vi "PSAS Data to text file (2).vi"(8 "Eixo":string, 9 "2nd column array":dbl[](array[numeric]), 10 "1st column array":dbl[](array[numeric]), 11 "Timestep":string) -> (2 "Data to text file":string)   [LabVIEW 2013]
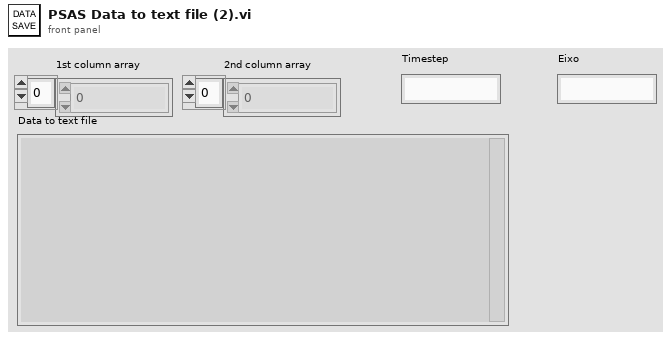
[diagram p1: front panel]
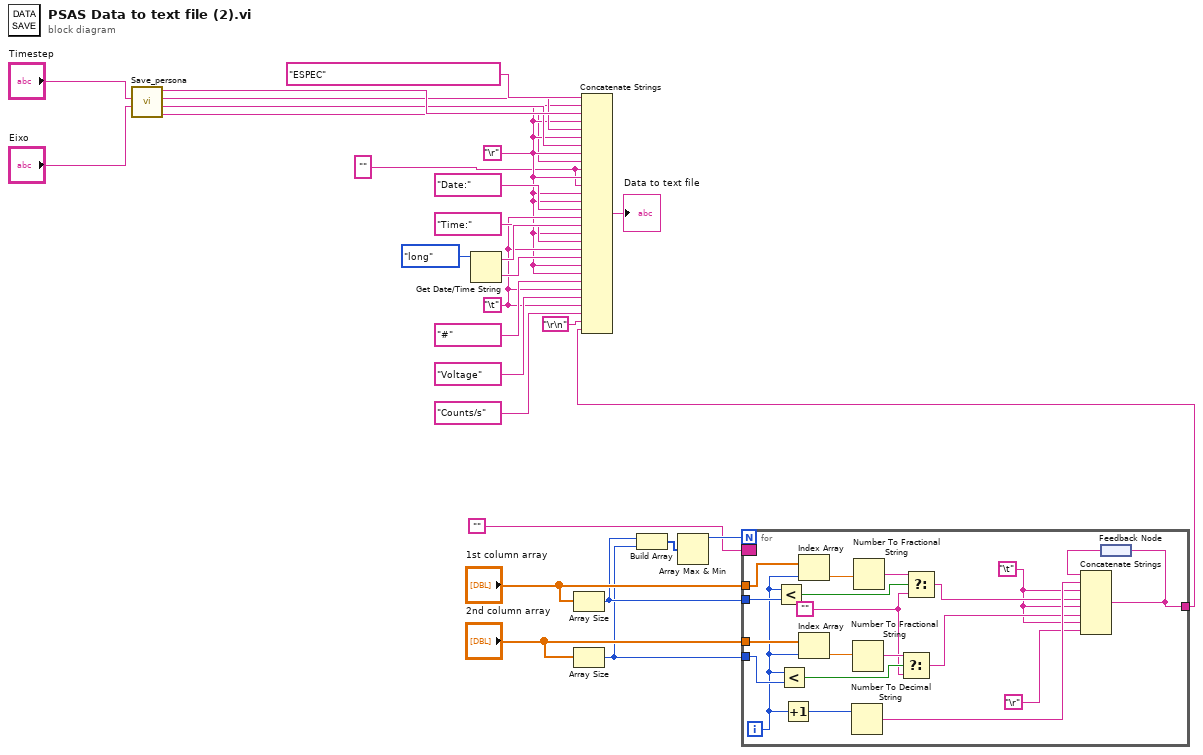
[diagram p0: block diagram]
diagram:
  w3 = "" ("string")
  w13 = "\t"
  w5 = "\r"
  n1 = call "Save_persona.vi"("Tipo de eixo dos XX"="Eixo", "Time Step:"="Timestep") -> ("Descrição:"=w4:string, "Tipo de eixo dos XX"=w6:string, "Time Step:"=w7:string, "Nome do utilizador:"=w8:string)  [unwired: 4 in]
  n2 = Get Date/Time String(date format (0)=enum16{"short", "long", "abbreviated"}."long") -> (date string=w28:string, time string=w25:string)  [unwired: 2 in]
  n3 = Array Size(array="1st column array") -> (size(s)=w15:i32)
  n4 = Array Size(array="2nd column array") -> (size(s)=w14:i32)
  n5 = Build Array(w15, w14) -> (w22:i32[])
  n6 = Array Max & Min(array=w22) -> (max value=w21:i32)  [unwired: 3 out]
  n7 = for {
    N: w21 -> [_]
    tunnel: "1st column array" -> [w44]
    tunnel: [w47] -> w10
    tunnel: "2nd column array" -> [w46]
    tunnel: w15 -> [w40]
    tunnel: w14 -> [w33]
    border: "" -> [_]
    i -> [w31]
    w29 = ""
    w30 = "\t"
    n8 = Less?(x=w31, y=w40) -> (x < y?=w39:bool)
    n9 = Less?(x=w31, y=w33) -> (x < y?=w32:bool)
    n10 = Increment(x=w31) -> (x+1=w36:i32)
    n11 = Index Array(array=w44, index=w31) -> (element=w41:dbl)
    n12 = Index Array(array=w46, index=w31) -> (element=w45:dbl)
    n13 = Number To Decimal String(number=w36) -> (decimal integer string=w43:string)  [unwired: 1 in]
    n14 = Number To Fractional String(number=w45) -> (F-format string=w34:string)  [unwired: 3 in]
    n15 = Number To Fractional String(number=w41) -> (F-format string=w38:string)  [unwired: 3 in]
    n16 = Select(t=w34, s=w32, f=w29) -> (s? t:f=w35:string)
    n17 = Select(t=w38, s=w39, f=w29) -> (s? t:f=w37:string)
    n18 = feedback #1() -> (w48:string)
    n19 = Concatenate Strings(w48, w43, w30, w37, w30, w35, w30, "\r") -> (w47:string)
    n20 = feedback-in #1(w47) -> ()
  }
  n21 = Concatenate Strings("ESPEC", w5, w8, w5, w7, w5, w6, w5, w4, w3, w5, w3, w5, w5, "Date:", w13, w28, w5, "Time:", w13, w25, w5, w5, "#", w13, "Voltage", w13, "Counts/s", "\r\n", w10) -> (→"Data to text file":string)
